vi "Measuare Leak dut - chamber.vi"(7 "changed or first call?":bool, 8 "error in (no error)":errorcluster, 11 "Stand in":refnum<class "Stand.lvclass">) -> (0 "error in (no error) 2":errorcluster, 3 "Stand in 2":refnum<class "Stand.lvclass">)   [LabVIEW 2019, in "Stand.lvclass"]
uses:
  Stand.lvclass
  D:/GIT H4000/H4000/src/Device_class/Device.lvclass
  TypeDef/Direction.ctl
  Device_class/Device.lvclass/Device.ctl
  Stand.lvclass/Stand.ctl
  AI_class/AI.lvclass/AI.ctl
  AnalogComparator_class/AnalogComparator.lvclass/AnalogComparator.ctl
  Valve DIR.ctl
  NeedleValve_class/Cmd.ctl
  0354d74f-2998-4c32-b28e-22161266d32a.vi
  subvis/FastForward.vi
  Get U max Haskel.vi
  Get Accuracy.vi
  DoValve.vi
  AnalogComparator_class/GetStatus.vi
  DoValve.vi/e7d2c9dc-ba67-4685-b926-bcce34aa2778.vi
  DoValve.vi/628819af-fd07-4303-9780-3ddd467101db.vi
  Global/Global Constant.vi
  <vilib>/addons/_JKI.lib/FPGA_Basic_Components/Counter JKI_FPGA.vi
  <vilib>/addons/_JKI.lib/FPGA_Basic_Components/Counter_32bit JKI_FPGA.vi
  Const All Valve.vi
  FPGA_API_class/FPGA API.lvclass
  NeedleValve_class/NeedleValve.lvclass
  AI_class/AI.lvclass
  Device_class/Device.lvclass
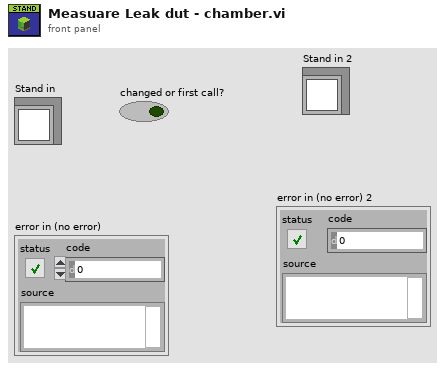
[diagram p1: front panel]
types:
  T1 = typedef "Direction.ctl" = enum8{"DUT", "Chamber"}
  T2 = typedef "Valve DIR.ctl" = enum16{"Air Valves: Open (DUT Filling)", "Air Valves: Open (Chamber Filling)", "Air Valves: Open (Pump Pressure DUT)", "Air Valves: Open (Pump Pressure Chamber)", "Air Valves: Open (Haskel Pressure DUT)", "Air Valves: Open (Haskel Pressure Chamber)", "Air Valves: Open (Slow Release DUT)", "Air Valves: Open (Slow Release Chamber)", "Air Valves: Open (Fast Release DUT)", "Air Valves: Open (Fast Release Chamber)", "Air Valves: Open (Emergency Release DUT and Chamber)", "Air Valves: Leak Hi (Chamber)", "Air Valves: Leak Hi (DUT)", "Air Valves: Backpressure (Chamber)", "Air Valves: Backpressure (DUT)", "Air Valves: Fully Closed", "Air Valves: Open 33.7"}
  T3 = typedef "NeedleValve.lvclass/Cmd.ctl" = enum16{"Open", "Close", "Stop", "Prep open"}
  T4 = typedef "AI_Data.ctl" = cluster{"Stat Data":T5, "OutOfRangeMax":bool, "OutOfRangeMin":bool, "HIHI":bool, "HI":bool, "LO":bool, "LOLO":bool}
  T5 = typedef "AI Statistics Data.ctl" = cluster{"raw mean":dbl, "scl mean":dbl, "raw mean 1Hz":dbl, "scl mean 1Hz":dbl}
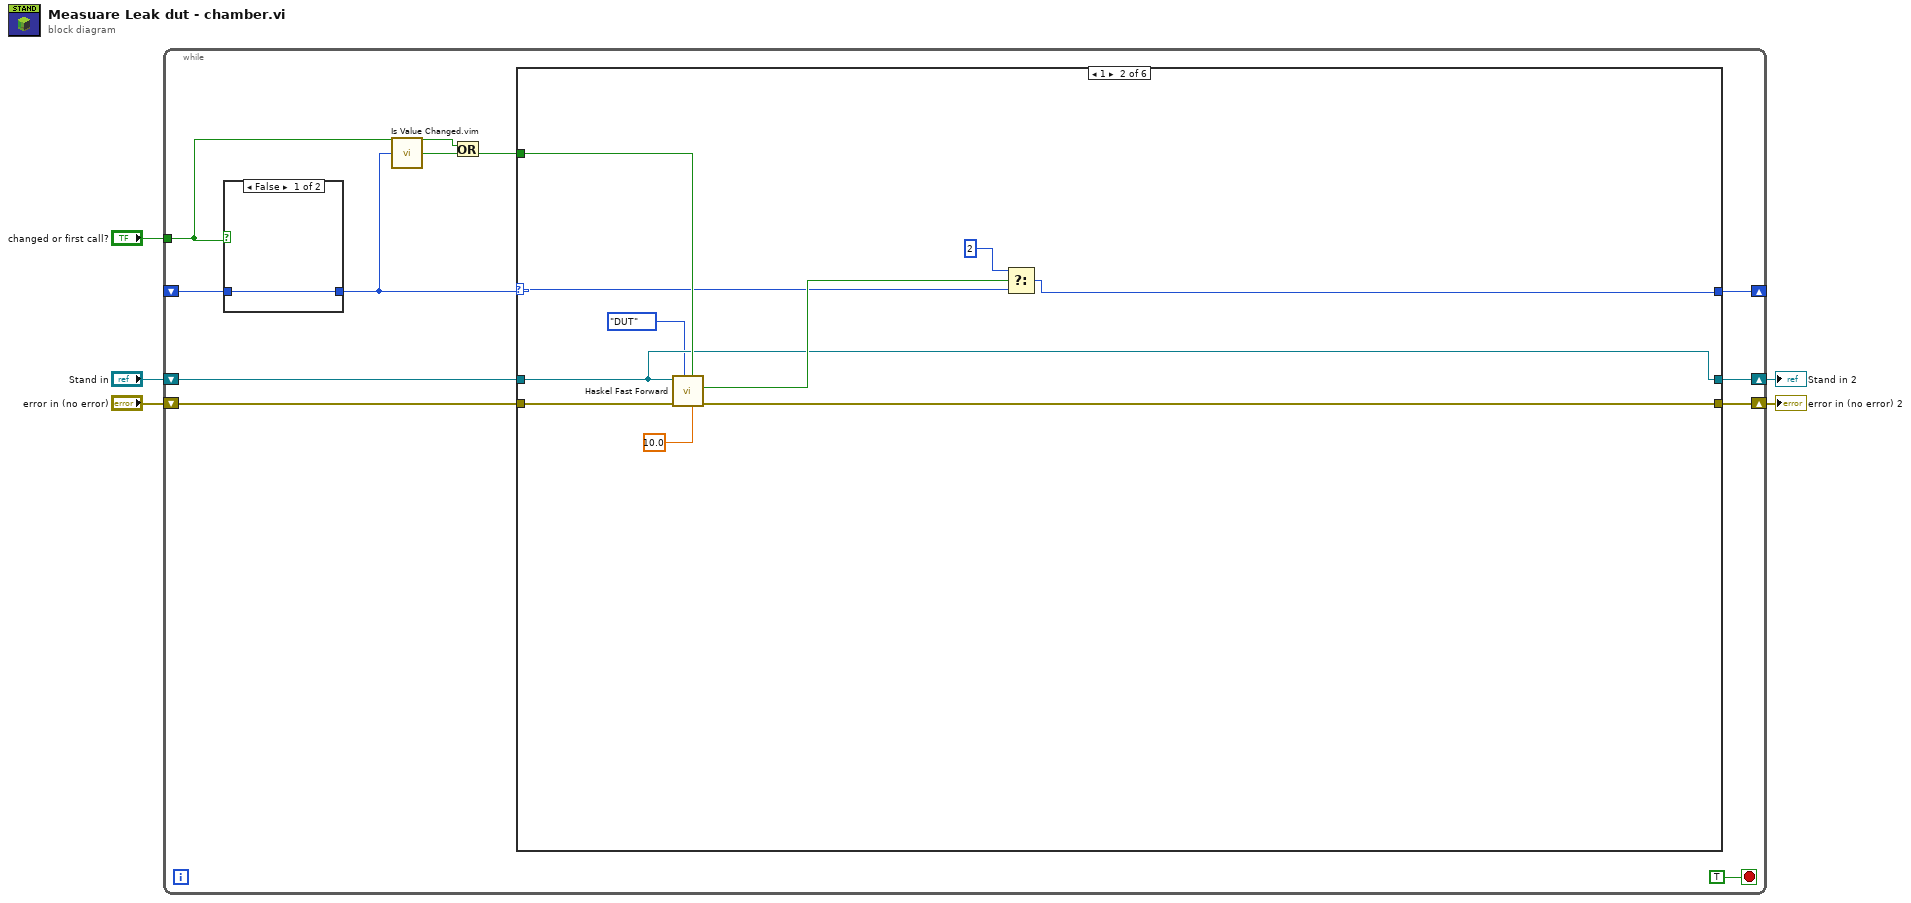
[diagram p0: block diagram]
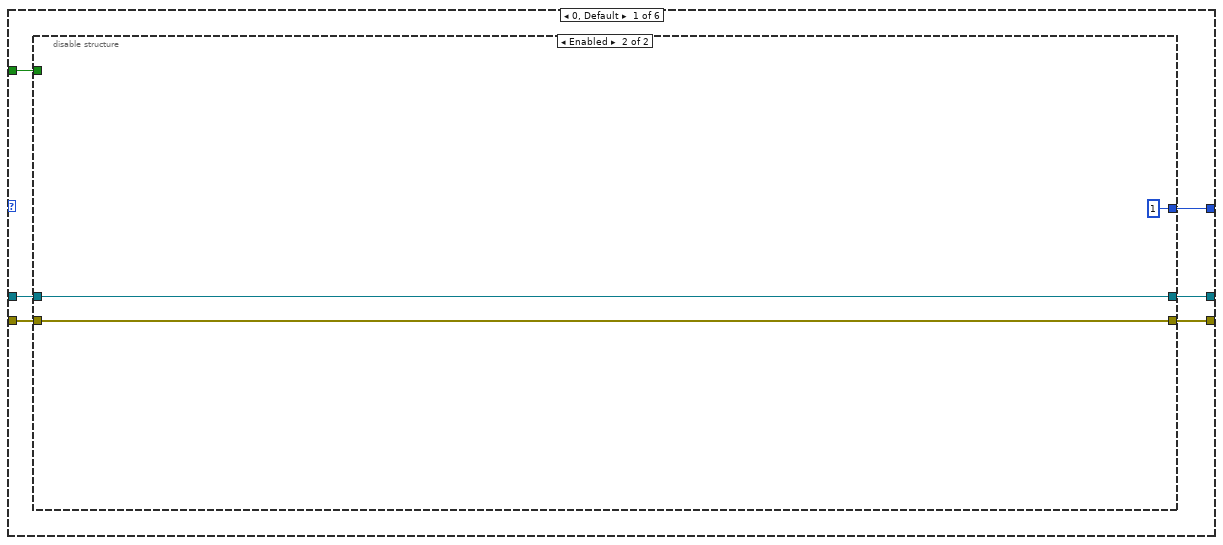
[diagram p3: hidden frame]
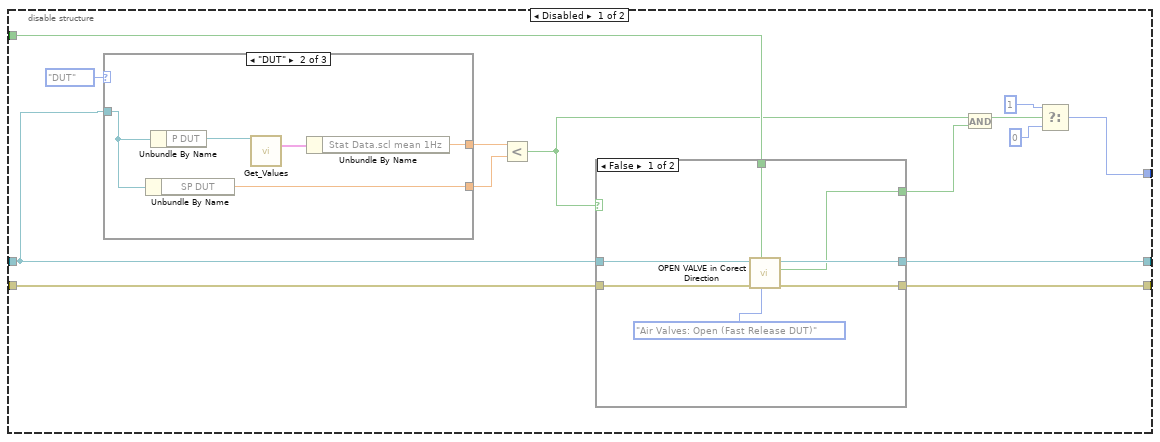
[diagram p4: hidden frame]
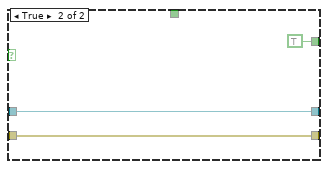
[diagram p5: hidden frame]
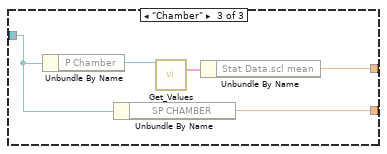
[diagram p7: hidden frame]
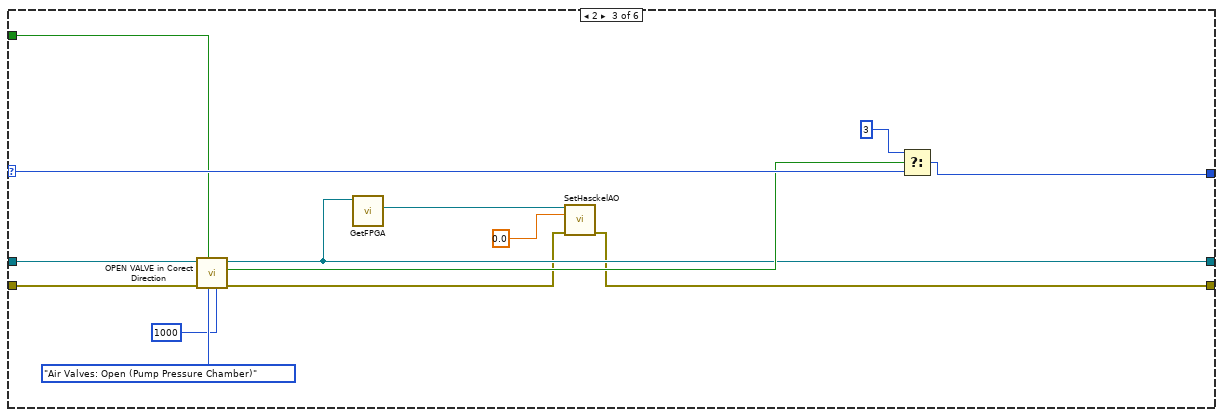
[diagram p8: hidden frame]
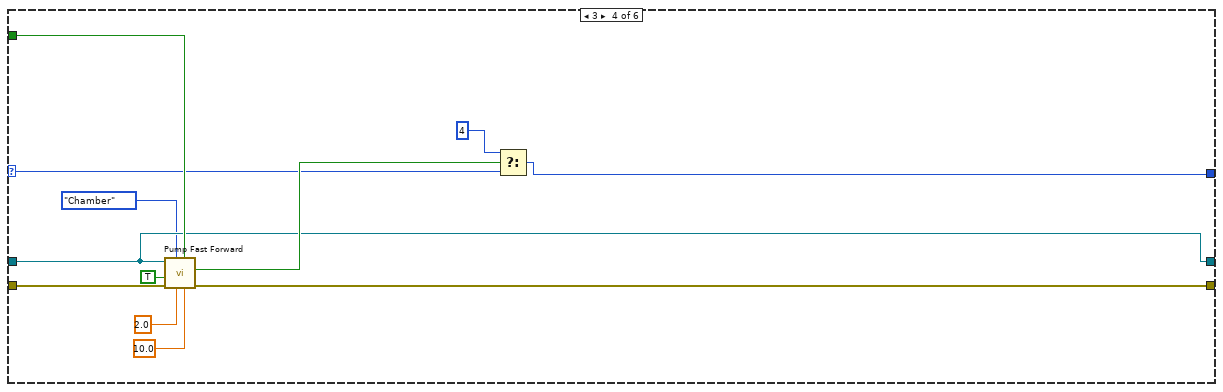
[diagram p9: hidden frame]
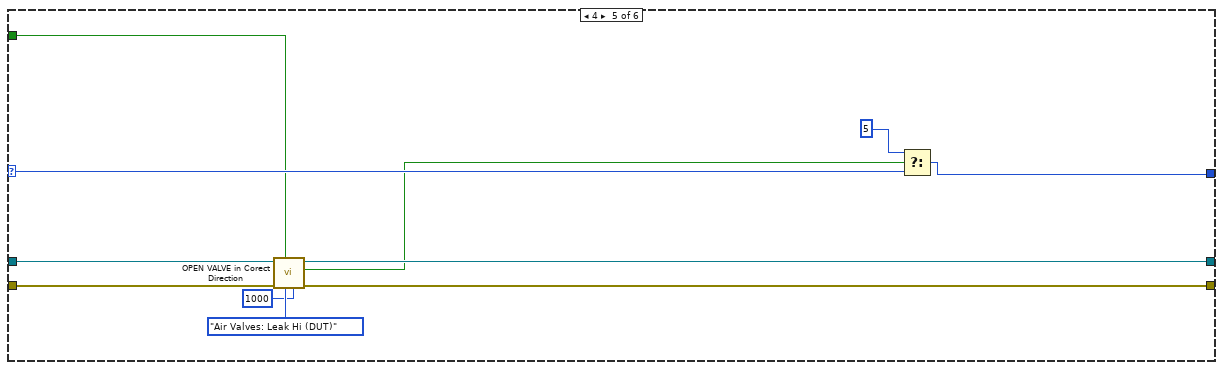
[diagram p10: hidden frame]
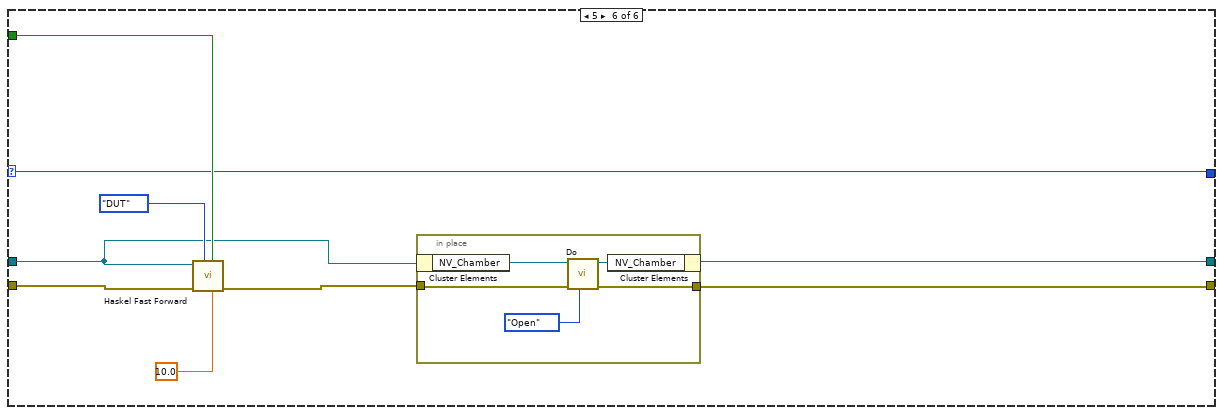
[diagram p11: hidden frame]
diagram:
  n1 = while {
    shift-right: [w9] -> _
    shift-left: _ -> [w12]
    shift-right: [w8] -> w2
    shift-left: "Stand in" -> [w15]
    shift-right: [w10] -> w1
    shift-left: "error in (no error)" -> [w14]
    tunnel: "changed or first call?" -> [w6]
    stop <- TRUE stop-if-true
    n2 = case shown="False" w6 {
      tunnel: w12 -> [w17 _]
      tunnel: [w17 _] -> w11
      frame False {
      }
      frame True {
      }
    }
    n3 = call "Is Value Changed.vim"("value"=w11) -> ("changed or first call?"=w13:bool)
    n4 = Or(x=w6, y=w13) -> (x .or. y?=w7:bool)
    n5 = case shown="1" w11 {
      selector: w11 -> [_ w66 w84 w92 w107 w109]
      tunnel: w15 -> [w22 w63 w81 w89 w104 w112]
      tunnel: w14 -> [w20 w70 w79 w96 w103 w116]
      tunnel: w7 -> [w19 w69 w80 w95 w98 w115]
      tunnel: [w21 w67 w72 w93 w101 w111] -> w10
      tunnel: [w18 w65 w83 w91 w106 w109] -> w9
      tunnel: [w23 w63 w75 w89 w100 w110] -> w8
      frame 0, Default {
        n6 = disable-structure shown="Enabled" {
          disable-tunnel: [w37 w59] -> w23
          disable-tunnel: w22 -> [w36 w59]
          disable-tunnel: [w32 w58] -> w21
          disable-tunnel: w20 -> [w31 w58]
          disable-tunnel: w19 -> [w30 _]
          disable-tunnel: [w26 1 ("t")] -> w18
          frame Disabled {
            n7 = case shown="\"DUT\"" Direction."DUT" ("Direction") {
              tunnel: [_ w52 w57] -> w34
              tunnel: [_ w50 w55] -> w33
              tunnel: w36 -> [_ w49 w54]
              frame "DUT", Default {
              }
              frame "DUT" {
                n8 = Unbundle By Name(w49) -> ("SP DUT"=w50:dbl)
                n9 = Unbundle By Name(w49) -> ("P DUT"=w48:refnum<class "AI.lvclass">)
                n10 = call "Get_Values.vi"("reference in"=w48) -> ("Data"=w51:T4)  [unwired: 14 in]
                n11 = Unbundle By Name(w51) -> ("Stat Data.scl mean 1Hz"=w52:dbl)
              }
              frame "Chamber" {
                n12 = Unbundle By Name(w54) -> ("P Chamber"=w53:refnum<class "AI.lvclass">)
                n13 = Unbundle By Name(w54) -> ("SP CHAMBER"=w55:dbl)
                n14 = call "Get_Values.vi"("reference in"=w53) -> ("Data"=w56:T4)  [unwired: 14 in]
                n15 = Unbundle By Name(w56) -> ("Stat Data.scl mean"=w57:dbl)
              }
            }
            n16 = Less?(x=w34, y=w33) -> (x < y?=w29:bool)
            n17 = case shown="False" w29 {
              tunnel: [w43 w47] -> w37
              tunnel: w36 -> [w42 w47]
              tunnel: [w40 w46] -> w32
              tunnel: w31 -> [w41 w46]
              tunnel: w30 -> [w39 _]
              tunnel: [w38 TRUE ("Done")] -> w24
              frame False {
                n18 = call "OPEN VALVE in Corect Direction.vi"("Valve DIR"=Valve_DIR."Air Valves: Open (Fast Release DUT)", "changed or first call?"=w39, "error in (no error)"=w41, "Stand in"=w42) -> ("error out"=w40:errorcluster, "Done"=w38:bool, "Stand out"=w43:refnum<class "Stand.lvclass">)  [unwired: 5 in]
              }
              frame True {
              }
            }
            n19 = And(x=w29, y=w24) -> (x .and. y?=w25:bool)
            n20 = Select(t=1, s=w25, f=0 ("t")) -> (s? t:f=w26:i32)
          }
          frame Enabled {
          }
        }
      }
      frame 1 {
        n21 = call "Haskel Fast Forward.vi"("Time Target (s)"=10.0, "Init"=w69, "Direction"=Direction."DUT", "error in (no error)"=w70, "Stand in"=w63) -> ("error out"=w67:errorcluster, "Done"=w68:bool)  [unwired: 5 in]
        n22 = Select(t=2, s=w68, f=w66) -> (s? t:f=w65:i32)
      }
      frame 2 {
        n23 = call "OPEN VALVE in Corect Direction.vi"("time after close"=u32 1000, "Valve DIR"=Valve_DIR."Air Valves: Open (Pump Pressure Chamber)", "changed or first call?"=w80, "error in (no error)"=w79, "Stand in"=w81) -> ("error out"=w73:errorcluster, "Done"=w77:bool, "Stand out"=w75:refnum<class "Stand.lvclass">)  [unwired: 4 in]
        n24 = call "GetFPGA.vi"("Device in"=w75) -> ("FPGA API.lvclass"=w76:refnum<class "FPGA API.lvclass">)  [unwired: 10 in]
        n25 = call-dynamic "SetHasckelAO.vi"("FPGA API in"=w76, "Haskel in"=0.0, "error in (no error)"=w73) -> ("error out"=w72:errorcluster)  [unwired: 11 in, 1 out]
        n26 = Select(t=3, s=w77, f=w84) -> (s? t:f=w83:i32)
      }
      frame 3 {
        n27 = call "Pump Fast Forward.vi"("Time Target (s)"=10.0, "Init"=w95, "percent"=2.0, "Direction"=Direction."Chamber", "error in (no error)"=w96, "Leak"=TRUE, "Stand in"=w89) -> ("error out"=w93:errorcluster, "Done"=w94:bool)  [unwired: 3 in]
        n28 = Select(t=4, s=w94, f=w92) -> (s? t:f=w91:i32)
      }
      frame 4 {
        n29 = call "OPEN VALVE in Corect Direction.vi"("time after close"=u32 1000, "Valve DIR"=Valve_DIR."Air Valves: Leak Hi (DUT)", "changed or first call?"=w98, "error in (no error)"=w103, "Stand in"=w104) -> ("error out"=w101:errorcluster, "Done"=w99:bool, "Stand out"=w100:refnum<class "Stand.lvclass">)  [unwired: 4 in]
        n30 = Select(t=5, s=w99, f=w107) -> (s? t:f=w106:i32)
      }
      frame 5 {
        n31 = call "Haskel Fast Forward.vi"("Time Target (s)"=10.0, "Init"=w115, "Direction"=Direction."DUT", "error in (no error)"=w116, "Stand in"=w112) -> ("error out"=w113:errorcluster)  [unwired: 5 in, 1 out]
        n32 = in-place {
          in-place-border: w113 -> [w119]
          in-place-border: [w118] -> w111
          n33 = in-place-cluster #1(w112) -> ("NV_Chamber"=w121:refnum<class "NeedleValve.lvclass">)
          n34 = call "Do.vi"("Cmd"=Cmd."Open", "error in (no error)"=w119, "NeedleValve in"=w121) -> ("error out"=w118:errorcluster, "NeedleValve out"=w120:refnum<class "NeedleValve.lvclass">)  [unwired: 7 in]
          n35 = in-place-cluster #1("NV_Chamber"=w120) -> (w110:refnum<class "Stand.lvclass">)
        }
      }
    }
  }
  "Stand in 2" <- w2
  "error in (no error) 2" <- w1
